vi "Get Buffers.vi"(11 "Plugin in":refnum<class "Plugin.lvclass">) -> (2 "Buffers":refnum<class "Buffers.lvclass">, 3 "Plugin out":refnum<class "Plugin.lvclass">)   [LabVIEW 2017, in "DSF Core.lvlib" / "Plugin.lvclass"]
uses:
  Plugin.lvclass
  Buffers/Buffers.lvclass
  Plugin.lvclass/Plugin.ctl
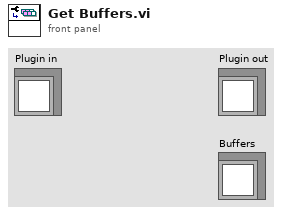
[diagram p1: front panel]
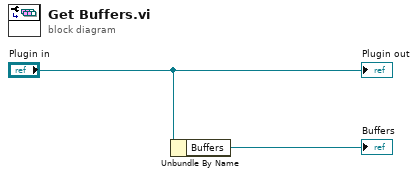
[diagram p0: block diagram]
diagram:
  n1 = Unbundle By Name("Plugin in") -> ("Buffers"=→"Buffers":refnum<class "Buffers.lvclass">)
  "Plugin out" <- "Plugin in"
